vi "Write Per-Site Ref Mic LUT INI File.vi"(0 "Per-Site Ref Mic LUT INI File Path":path, 5 "Per-Site Ref Mic LUT Data":string[][](table), 11 "error in (no error)":errorcluster, 12 "Delete Existing File?":bool) -> (15 "error out":errorcluster)   [LabVIEW 2020]
uses:
  <vilib>/Utility/config.llb/Write Key (I32).vi
  <vilib>/Utility/config.llb/Write Key (String).vi
  <vilib>/Utility/config.llb/NI_LVConfig.lvlib
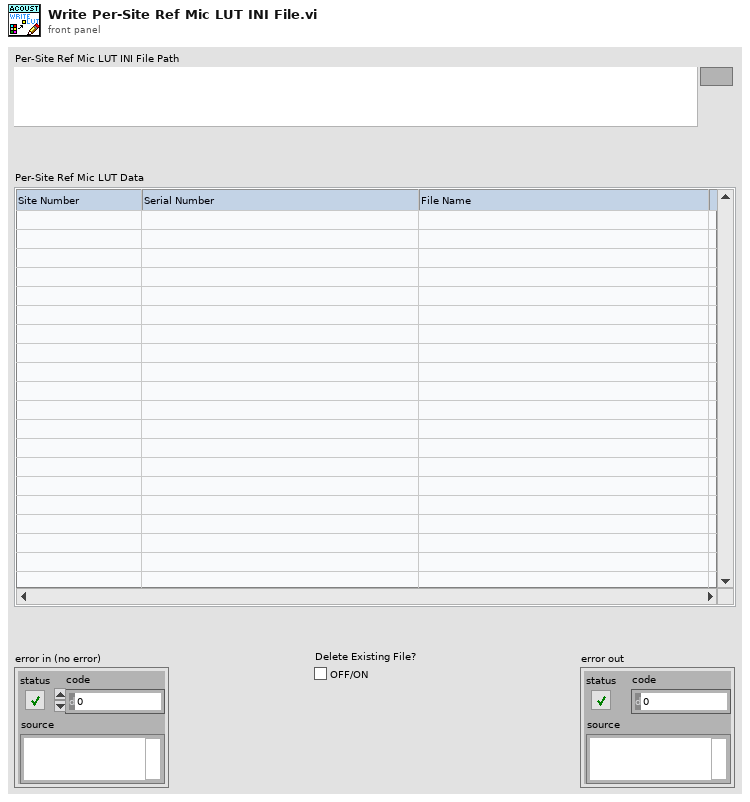
[diagram p1: front panel]
types:
  T1 = typedef "NI_LVConfig.lvlib/Config Data RefNum.ctl" = refnum<k1>
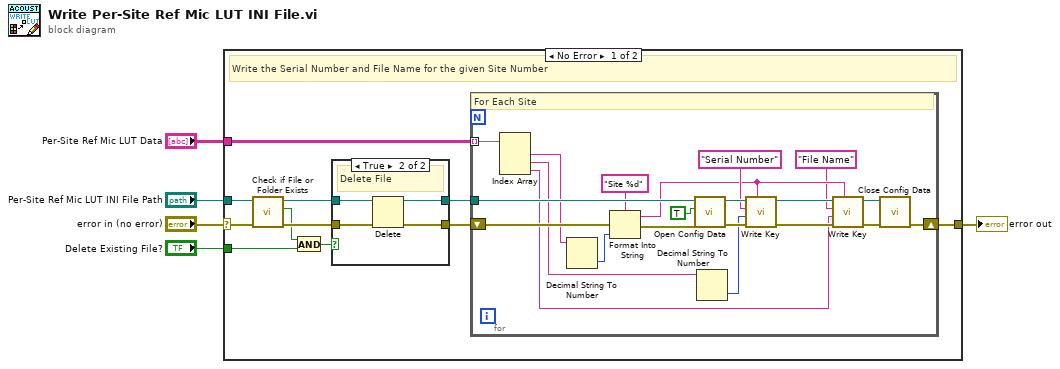
[diagram p0: block diagram]
diagram:
  n1 = case shown="No Error" "error in (no error)" {
    selector: "error in (no error)" -> [w14 w44]
    tunnel: [w16 w44] -> w5
    tunnel: "Per-Site Ref Mic LUT INI File Path" -> [w13 _]
    tunnel: "Per-Site Ref Mic LUT Data" -> [w15 _]
    tunnel: "Delete Existing File?" -> [w10 _]
    frame No Error {
      # "Write the Serial Number and File Name for the given Site Number"
      n2 = call <vilib>:"Check if File or Folder Exists.vi"("error in (no error)"=w14, "path"=w13) -> ("error out"=w11:errorcluster, "file or folder exists?"=w9:bool, "dup path"=w12:path)  [unwired: 7 in]
      n3 = And(x=w9, y=w10) -> (x .and. y?=w8:bool)
      n4 = case shown="True" w8 {
        tunnel: w12 -> [w18 w21]
        tunnel: w11 -> [w17 w22]
        tunnel: [w18 w20] -> w7
        tunnel: [w17 w19] -> w6
        frame False {
          # "Proceed Normally"
        }
        frame True {
          # "Delete File"
          n5 = Delete(path (use dialog)=w21, error in=w22) -> (deleted path=w20:path, error out=w19:errorcluster)  [unwired: 3 in, 1 out]
        }
      }
      n6 = for {
        tunnel: w7 -> [w43]
        shift-right: [w31] -> w16
        shift-left: w6 -> [w40]
        tunnel: w15 -> [w29] mode=indexing
        # "For Each Site"
        n7 = Index Array(array=w29) -> (element #1=w28:string, element #2=w25:string, element #3=w24:string)  [unwired: 3 in]
        n8 = Decimal String To Number(string=w28) -> (number=w27:i32)  [unwired: 2 in, 1 out]
        n9 = Format Into String(format string="Site %d", error in=w40, w27) -> (resulting string=w34:string, error out=w39:errorcluster)  [unwired: 1 in]
        n10 = call <vilib>:"Open Config Data.vi"("error in (no error)"=w39, "create file if necessary (T)"=TRUE, "configuration file path"=w43) -> ("error out"=w42:errorcluster, "refnum"=w41:T1)  [unwired: 6 in, 1 out]
        n11 = Decimal String To Number(string=w25) -> (number=w23:i32)  [unwired: 2 in, 1 out]
        n12 = call-poly <vilib>:"Write Key.vi"("section"=w34, "error in (no error)"=w42, "value"=w23, "key"="Serial Number" ("section"), "refnum"=w41) -> ("error out"=w36:errorcluster, "refnum out"=w35:T1)  [unwired: 4 in, 1 out]
        n13 = call-poly <vilib>:"Write Key.vi"("section"=w34, "error in (no error)"=w36, "value"=w24, "key"="File Name" ("section"), "refnum"=w35) -> ("error out"=w32:errorcluster, "refnum out"=w30:T1)  [unwired: 4 in, 1 out]
        n14 = call <vilib>:"Close Config Data.vi"("error in (no error)"=w32, "refnum"=w30) -> ("error out"=w31:errorcluster)  [unwired: 8 in, 1 out]
      }
    }
    frame Error {
      # "Error case - Do Nothing"
    }
  }
  "error out" <- w5
